vi "Initialize Sensors.vi"(0 "UniCyRO_Host_Sim in":refnum<class "UniCyRO_Host_Sim.lvclass">, 1 "Sparkfun Atomic IMU out":refnum<class "Sparkfun Atomic IMU.lvclass">, 2 "Garmin GPS Series out":refnum<class "Garmin GPS Series.lvclass">, 3 "Honeywell Compass HMC6343":refnum<class "Honeywell Compass HMC6343.lvclass">, 4 "Hokuyo URG Series out":refnum<class "Hokuyo URG Series.lvclass">, 5 "error in (no error)":errorcluster, 7 "IMU Error":i32, 9 "GPS Error":i32, 11 "Compass Error":i32, 13 "LIDAR Error":i32) -> (14 "UniCyRO_Host_Sim out":refnum<class "UniCyRO_Host_Sim.lvclass">, 19 "error out":errorcluster)   [LabVIEW 2012, in "UniCyRO.lvlib" / "UniCyRO_Host_Sim.lvclass"]
uses:
  UniCyRO_Host_Sim.lvclass
  <instrlib>/Sparkfun Atomic IMU/HAIOL/Sparkfun Atomic IMU.lvclass
  <instrlib>/Hokuyo URG Series/HAIOL/Hokuyo URG Series.lvclass
  <instrlib>/Garmin GPS Series/HAIOL/Garmin GPS Series.lvclass
  <instrlib>/Honeywell Compass HMC6343/HAIOL/Honeywell Compass HMC6343.lvclass
  UniCyRO_Host_Sim.lvclass/UniCyRO_Host_Sim.ctl
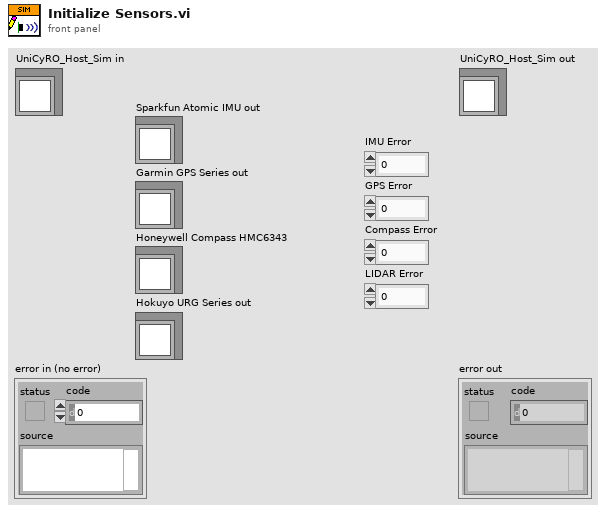
[diagram p1: front panel]
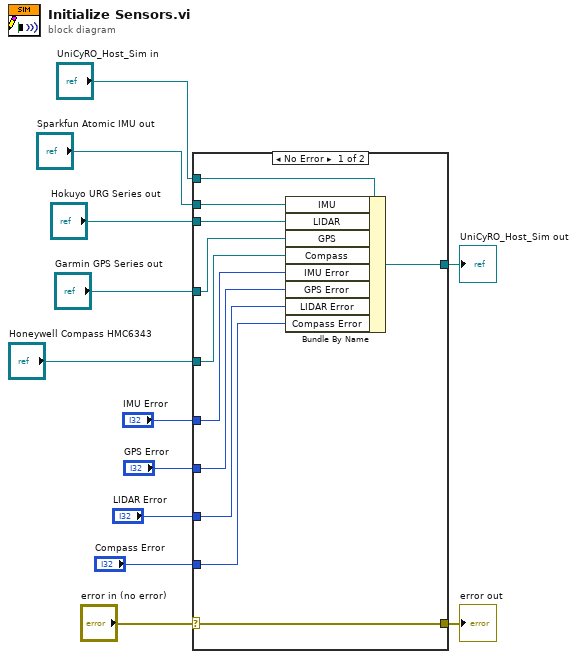
[diagram p0: block diagram]
diagram:
  n1 = case shown="No Error" "error in (no error)" {
    selector: "error in (no error)" -> [w23 w25]
    tunnel: [w23 w25] -> w11
    tunnel: [w21 w24] -> w9
    tunnel: "UniCyRO_Host_Sim in" -> [w22 w24]
    tunnel: "Sparkfun Atomic IMU out" -> [w20 _]
    tunnel: "Hokuyo URG Series out" -> [w19 _]
    tunnel: "Honeywell Compass HMC6343" -> [w18 _]
    tunnel: "Garmin GPS Series out" -> [w17 _]
    tunnel: "IMU Error" -> [w16 _]
    tunnel: "GPS Error" -> [w15 _]
    tunnel: "LIDAR Error" -> [w14 _]
    tunnel: "Compass Error" -> [w13 _]
    frame No Error {
      n2 = Bundle By Name(cluster=w22, "IMU"=w20, "LIDAR"=w19, "GPS"=w17, "Compass"=w18, "IMU Error"=w16, "GPS Error"=w15, "LIDAR Error"=w14, "Compass Error"=w13) -> (w21:refnum<class "UniCyRO_Host_Sim.lvclass">)
    }
    frame Error {
    }
  }
  "error out" <- w11
  "UniCyRO_Host_Sim out" <- w9
